vi "Begin.vi"(8 "error in":errorcluster) -> (0 "error out":errorcluster)   [LabVIEW 2018]
doc: "Called before other user functions, this VI can be used to open I/O refnums, load in file data, and do general program initialization. Notice that the <B>error out</B> terminal is simply used for data flow. Wiring it to other structures or subVIs ensures that this VI runs first."
uses:
  <vilib>/Rock Robotics/WPI/DriverStation/WPI_DriverStationRobotMode2.ctl
  <vilib>/Rock Robotics/WPI/Joystick/WPI_JoystickDeviceEnum.ctl
  <vilib>/Rock Robotics/SystemInterfaces/DIO/FPGA_DIOPWMChannel.ctl
  <vilib>/Rock Robotics/WPI/Solenoid/WPI_SolenoidChannel.ctl
  Robot Global Data.vi
  <vilib>/Rock Robotics/Network Tables/NT Write String Array.vi
  <vilib>/Rock Robotics/WPI/RobotDrive/WPI_RobotDriveOpen4MotorWithTalonSRX.vi
  <vilib>/Rock Robotics/WPI/RobotDrive/WPI_RobotDriveOpen4MotorWithVictorSP.vi
  <vilib>/Rock Robotics/WPI/RobotDrive/WPI_RobotDriveOpen2MotorWithVictorSP.vi
  <vilib>/Rock Robotics/WPI/Solenoid/WPI_SolenoidOpenDouble.vi
  <vilib>/Rock Robotics/SystemInterfaces/DIO/FPGA_DIOChannel.ctl
  <vilib>/Rock Robotics/WPI/MotorControl/WPI_MotorControlOpen SPARK.vi
  <vilib>/Rock Robotics/WPI/Counter/WPI_CounterDigitalInputToDigitalSource.vi
  <vilib>/Rock Robotics/WPI/Encoder/WPI_EncoderType.ctl
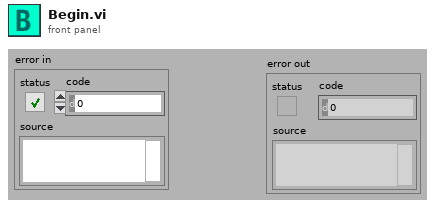
[diagram p1: front panel]
types:
  T1 = typedef "WPI_JoystickDeviceEnum.ctl" = enum16{"USB 0", "USB 1", "USB 2", "USB 3", "USB 4", "USB 5"}
  T2 = typedef "WPI_SolenoidChannel.ctl" = enum8{"Solenoid 0", "Solenoid 1", "Solenoid 2", "Solenoid 3", "Solenoid 4", "Solenoid 5", "Solenoid 6", "Solenoid 7", "Invalid"}
  T3 = typedef "FPGA_DIOPWMChannel.ctl" = enum8{"PWM 0", "PWM 1", "PWM 2", "PWM 3", "PWM 4", "PWM 5", "PWM 6", "PWM 7", "PWM 8", "PWM 9", "PWM MXP 0", "PWM MXP 1", "PWM MXP 2", "PWM MXP 3", "PWM MXP 4", "PWM MXP 5", "PWM MXP 6", "PWM MXP 7", "PWM MXP 8", "PWM MXP 9", "Invalid"}
  T4 = typedef "WPI_DriverStationRobotMode2.ctl" = enum16{"Autonomous Disabled", "Autonomous Enabled", "Teleop Disabled", "Teleop Enabled", "Disconnected", "Finish", "Test Disabled", "Test Enabled", "Emergency Stopped"}
  T5 = typedef "FPGA_DIOChannel.ctl" = enum8{"DIO 0", "DIO 1", "DIO 2", "DIO 3", "DIO 4", "DIO 5", "DIO 6", "DIO 7", "DIO 8", "DIO 9", "DIO MXP 0", "DIO MXP 1", "DIO MXP 2", "DIO MXP 3", "DIO MXP 4", "DIO MXP 5", "DIO MXP 6", "DIO MXP 7", "DIO MXP 8", "DIO MXP 9", "DIO MXP 10", "DIO MXP 11", "DIO MXP 12", "DIO MXP 13", "DIO MXP 14", "DIO MXP 15", "SPI Port CS1", "SPI Port CS2", "SPI Port CS3", "SPI Port MISO", "SPI Port MOSI", "Invalid"}
  T6 = typedef "WPI_CompressorDevRef.ctl" = cluster{"DevStatus":errorcluster, "Pneumatics Control Module":u8}
  T7 = typedef "WPI_DigitalInputDevRef.ctl" = cluster{"DevStatus":errorcluster, "DIO Channel":T5}
  T8 = typedef "WPI_SolenoidDevRef.ctl" = cluster{"DevStatus":errorcluster, "Pneumatics Control Module":u8, "Forward Solenoid Channel":T2, "Reverse Solenoid Channel":T2}
  T9 = typedef "WPI_MotorControlDeviceRef.ctl" = cluster{"DeviceStatus":errorcluster, "Type":T10, "PWM":cluster{"PWM Channel":T3, "DeadBand":T11}, "CAN":cluster{"Device Number":u8, "SetOutput VI Ref":variant, "GetOutput VI Ref":variant, "Enable VI Ref":variant, "Disable VI Ref":variant, "Data":variant}, "Invert":bool, "DIO PWM":cluster{"PWM \"Enable\" Channel":T3, "DIOChannel":T5, "PWM Rate":dbl}}
  T10 = typedef "WPI_MotorControlType.ctl" = enum16{"PWM", "CAN", "DIO PWM"}
  T11 = typedef "WPI_PWMDeadband.ctl" = cluster{"Name":string, "maxPositivePwm":i32, "minPositivePwm":i32, "centerPwm":i32, "maxNegativePwm":i32, "minNegativePwm":i32, "angularRange":u16}
  T12 = typedef "WPI_JoystickDevRef.ctl" = cluster{"Device":T1}
  T13 = typedef "WPI_RobotDriveDevRef.ctl" = cluster{"DevStatus":errorcluster, "Motors[]":T9[], "Square Inputs":bool, "Max Output":dbl}
  T14 = typedef "WPI_EncoderType.ctl" = enum16{"1x", "2x", "4x"}
  T15 = typedef "FPGA_CounterEncoderSourceConvertionLVSourceType.ctl" = cluster{"DevStatus":errorcluster, "AnalogTriggerMode?":bool, "DigitalMode":cluster{"DIO Channel":T16}, "AnalogTriggerMode":cluster{"AnalogTriggerIndex":T17, "OutputType":T18}}
  T16 = typedef "FPGA_DIODigitalSourceChannel.ctl" = enum8{"DIO 0", "DIO 1", "DIO 2", "DIO 3", "DIO 4", "DIO 5", "DIO 6", "DIO 7", "DIO 8", "DIO 9", "DIO MXP 0", "DIO MXP 1", "DIO MXP 2", "DIO MXP 3", "DIO MXP 4", "DIO MXP 5", "DIO MXP 6", "DIO MXP 7", "DIO MXP 8", "DIO MXP 9", "DIO MXP 10", "DIO MXP 11", "DIO MXP 12", "DIO MXP 13", "DIO MXP 14", "DIO MXP 15", "SPI Port CS1", "SPI Port CS2", "SPI Port CS3", "SPI Port MISO", "SPI Port MOSI", "Disabled"}
  T17 = typedef "FPGA_AnalogTriggerIndex.ctl" = enum8{"Trig 0", "Trig 1", "Trig 2", "Trig 3", "Trig 4", "Trig 5", "Trig 6", "Trig 7", "Invalid"}
  T18 = typedef "FPGA_AnalogTriggerOutType.ctl" = enum16{"InWindow", "TriggerState", "Rising", "Falling"}
  T19 = typedef "WPI_EncoderDevRef.ctl" = cluster{"DevStatus":errorcluster, "EncoderIndex":T20, "CounterIndex":T21, "DistancePerCount":dbl, "Decoding Type":T14}
  T20 = typedef "FPGA_EncoderIdx.ctl" = enum8{"Enc 0", "Enc 1", "Enc 2", "Enc 3", "Enc 4", "Enc 5", "Enc 6", "Enc 7", "Invalid"}
  T21 = typedef "FPGA_CounterCtrSystemIndex.ctl" = enum8{"Ctr 0", "Ctr 1", "Ctr 2", "Ctr 3", "Ctr 4", "Ctr 5", "Ctr 6", "Ctr 7", "Invalid"}
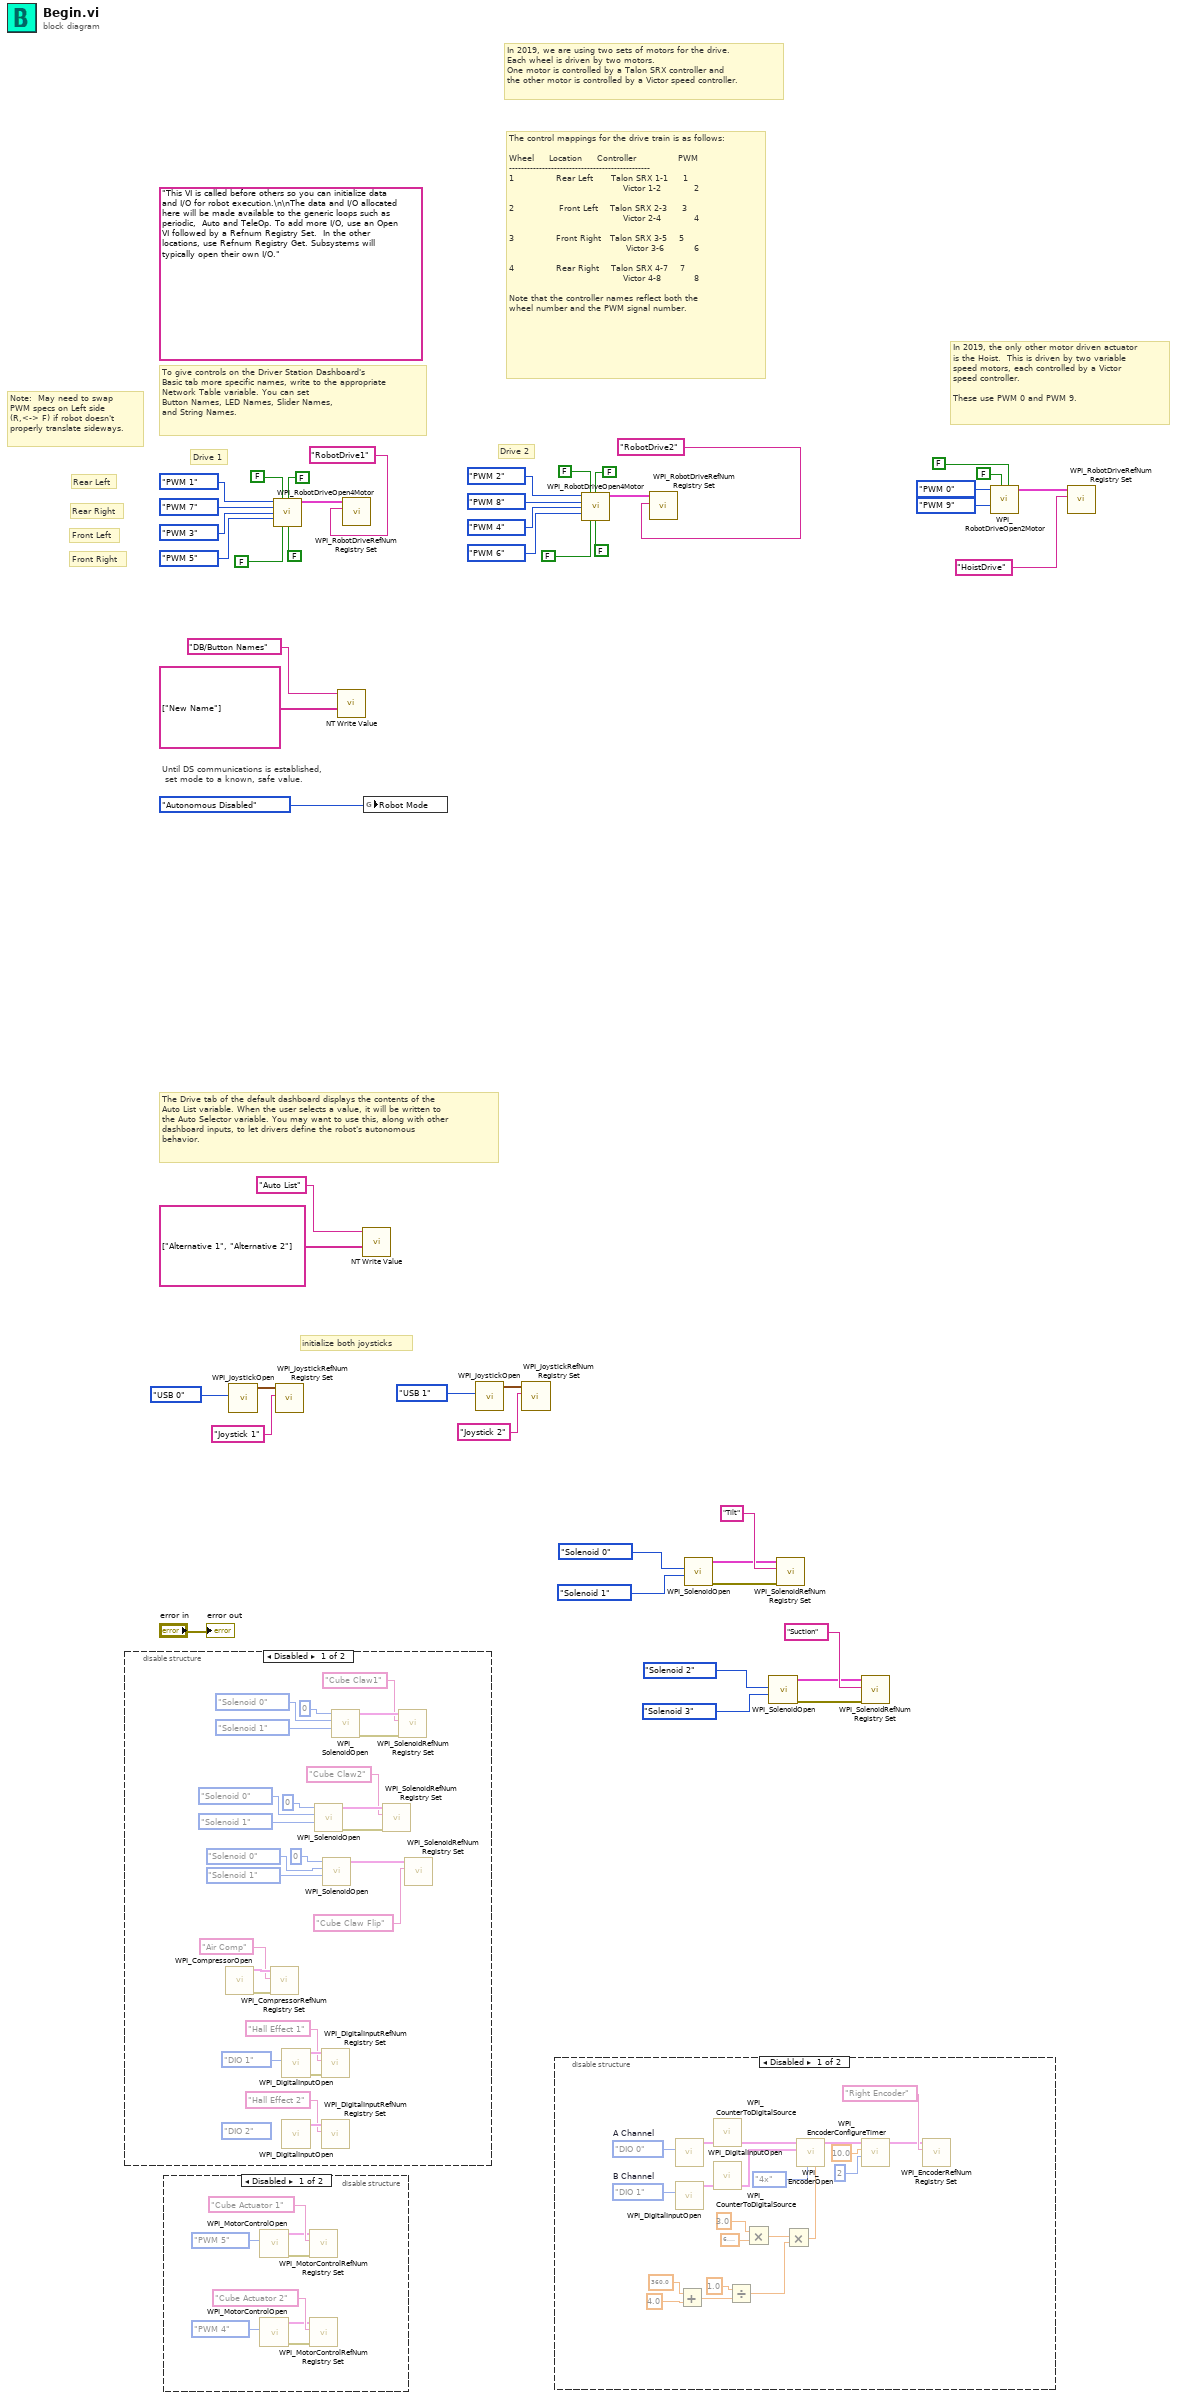
[diagram p0: block diagram]
diagram:
  (unwired) "This VI is called before others so you can initialize data and I/O for robot execution.\n\nThe data and I/O allocated here will be made available to the generic loops such as periodic,  Auto and TeleOp. To add more I/O, use an Open VI followed by a Refnum Registry Set.  In the other locations, use Refnum Registry Get. Subsystems will typically open their own I/O."
  # "In 2019, the only other motor driven actuator\nis the Hoist.  This is driven by two variable\nspeed motors, each controlled by a Victor \nspeed controller.\n\nThese use PWM 0 and PWM 9."
  # "Note:  May need to swap\nPWM specs on Left side \n(R,<-> F) if robot doesn't\nproperly translate sideways."
  # "Front Right"
  # "Front Left"
  # "Rear Left"
  # "Rear Right"
  # "The control mappings for the drive train is as follows:\n\nWheel     Location     Controller              PWM\n-----------------------------------------------\n1              Rear Left      Talon SRX 1-1     1\n                                      Victor 1-2           2\n\n2               Front Left    Talon SRX 2-3     3\n                                      Victor 2-4           4\n\n3              Front Right   Talon SRX 3-5    5\n                                       Victor 3-6          6\n\n4              Rear Right    Talon SRX 4-7    7\n                                      Victor 4-8           8\n\nNote that the controller names reflect both the\nwheel number and the PWM signal number."
  # "Drive 2"
  # "In 2019, we are using two sets of motors for the drive.\nEach wheel is driven by two motors.\nOne motor is controlled by a Talon SRX controller and \nthe other motor is controlled by a Victor speed controller."
  # "Drive 1"
  # "The Drive tab of the default dashboard displays the contents of the\nAuto List variable. When the user selects a value, it will be written to\nthe Auto Selector variable. You may want to use this, along with other\ndashboard inputs, to let drivers define the robot's autonomous\nbehavior."
  # "To give controls on the Driver Station Dashboard's\nBasic tab more specific names, write to the appropriate\nNetwork Table variable. You can set\nButton Names, LED Names, Slider Names,\nand String Names."
  # "initialize both joysticks"
  # "Until DS communications is established,\n set mode to a known, safe value."
  n1 = disable-structure shown="Disabled" {
    frame Disabled {
      (unwired) FPGA_DIOChannel."DIO 2" ("DIO Channel")
      n2 = call <vilib>:"WPI_CompressorOpen.vi"() -> ("CompressorDevRef"=w73:T6, "error out"=w74:errorcluster)  [unwired: 14 in]
      n3 = call <vilib>:"WPI_CompressorRefNum Registry Set.vi"("error in (no error)"=w74, "refnum name"="Air Comp", "CompressorDevRef"=w73) -> ()  [unwired: 7 in, 2 out]
      n4 = call <vilib>:"WPI_DigitalInputOpen.vi"("DIO Channel"=FPGA_DIOChannel."DIO 1") -> ("error out"=w49:errorcluster, "DigitalInputDevRef"=w54:T7)  [unwired: 9 in]
      n5 = call <vilib>:"WPI_DigitalInputOpen.vi"() -> ("DigitalInputDevRef"=w51:T7)  [unwired: 10 in, 1 out]
      n6 = call-poly <vilib>:"WPI_SolenoidOpen.vi"("Reverse Solenoid Channel"=WPI_SolenoidChannel."Solenoid 1", "Forward Solenoid Channel"=WPI_SolenoidChannel."Solenoid 0", "Pneumatics Control Module (0)"=u8 0) -> ("error out"=w64:errorcluster, "SolenoidDevRef"=w65:T8)  [unwired: 7 in]
      n7 = call <vilib>:"WPI_DigitalInputRefNum Registry Set.vi"("error in (no error)"=w49, "refnum name"="Hall Effect 1", "DigitalInputDevRef"=w54) -> ()  [unwired: 7 in, 2 out]
      n8 = call <vilib>:"WPI_DigitalInputRefNum Registry Set.vi"("refnum name"="Hall Effect 2", "DigitalInputDevRef"=w51) -> ()  [unwired: 8 in, 2 out]
      n9 = call-poly <vilib>:"WPI_SolenoidOpen.vi"("Reverse Solenoid Channel"=WPI_SolenoidChannel."Solenoid 1", "Forward Solenoid Channel"=WPI_SolenoidChannel."Solenoid 0", "Pneumatics Control Module (0)"=u8 0) -> ("SolenoidDevRef"=w59:T8)  [unwired: 7 in, 1 out]
      n10 = call-poly <vilib>:"WPI_SolenoidOpen.vi"("Reverse Solenoid Channel"=WPI_SolenoidChannel."Solenoid 1", "Forward Solenoid Channel"=WPI_SolenoidChannel."Solenoid 0", "Pneumatics Control Module (0)"=u8 0) -> ("error out"=w70:errorcluster, "SolenoidDevRef"=w71:T8)  [unwired: 7 in]
      n11 = call <vilib>:"WPI_SolenoidRefNum Registry Set.vi"("error in (no error)"=w64, "refnum name"="Cube Claw2", "SolenoidDevRef"=w65) -> ()  [unwired: 7 in, 2 out]
      n12 = call <vilib>:"WPI_SolenoidRefNum Registry Set.vi"("error in (no error)"=w70, "refnum name"="Cube Claw1", "SolenoidDevRef"=w71) -> ()  [unwired: 7 in, 2 out]
      n13 = call <vilib>:"WPI_SolenoidRefNum Registry Set.vi"("refnum name"="Cube Claw Flip", "SolenoidDevRef"=w59) -> ()  [unwired: 8 in, 2 out]
    }
    frame Enabled {
    }
  }
  n14 = disable-structure shown="Disabled" {
    frame Disabled {
      n15 = call-poly <vilib>:"WPI_MotorControlOpen.vi"("PWM Channel"=FPGA_DIOPWMChannel."PWM 5") -> ("error out"=w78:errorcluster, "MotorControlDeviceRef"=w77:T9)  [unwired: 9 in]
      n16 = call-poly <vilib>:"WPI_MotorControlOpen.vi"("PWM Channel"=FPGA_DIOPWMChannel."PWM 4") -> ("error out"=w80:errorcluster, "MotorControlDeviceRef"=w81:T9)  [unwired: 9 in]
      n17 = call <vilib>:"WPI_MotorControlRefNum Registry Set.vi"("error in (no error)"=w78, "refnum name"="Cube Actuator 1", "MotorControlDevRef"=w77) -> ()  [unwired: 7 in, 2 out]
      n18 = call <vilib>:"WPI_MotorControlRefNum Registry Set.vi"("error in (no error)"=w80, "refnum name"="Cube Actuator 2", "MotorControlDevRef"=w81) -> ()  [unwired: 7 in, 2 out]
    }
    frame Enabled {
    }
  }
  n19 = call <vilib>:"WPI_JoystickOpen.vi"("JoystickDevice"=WPI_JoystickDeviceEnum."USB 0") -> ("JoystickDevRef"=w46:T12)  [unwired: 10 in]
  n20 = call-poly <vilib>:"WPI_RobotDriveOpen4Motor.vi"("Rear Left Motor"=FPGA_DIOPWMChannel."PWM 1", "Rear Left Motor Inverted"=FALSE, "Rear Right Motor Inverted"=FALSE, "Rear Right Motor"=FPGA_DIOPWMChannel."PWM 7", "Front Left Motor"=FPGA_DIOPWMChannel."PWM 3", "Front Right Motor"=FPGA_DIOPWMChannel."PWM 5", "Front Left Motor Inverted"=FALSE, "Front Right Motor Inverted"=FALSE) -> ("RobotDriveDevRef"=w38:T13)  [unwired: 6 in, 1 out]
  n21 = call <vilib>:"WPI_JoystickRefNum Registry Set.vi"("refnum name"="Joystick 1", "JoystickDevRef"=w46) -> ()  [unwired: 8 in, 2 out]
  n22 = call-poly <vilib>:"NT Write Value.vi"("String Array"=string[] ["New Name"], "Name"="DB/Button Names") -> ()  [unwired: 9 in, 1 out]
  n23 = call <vilib>:"WPI_RobotDriveRefNum Registry Set.vi"("refnum name"="RobotDrive1", "RobotDriveDevRef"=w38) -> ()  [unwired: 8 in, 2 out]
  n24 = call-poly <vilib>:"NT Write Value.vi"("String Array"=string[] ["Alternative 1", "Alternative 2"], "Name"="Auto List") -> ()  [unwired: 9 in, 1 out]
  n25 = global write "Robot Global Data.vi" "Robot Mode"(WPI_DriverStationRobotMode2."Autonomous Disabled" ("Robot Mode")) -> ()
  n26 = call <vilib>:"WPI_JoystickOpen.vi"("JoystickDevice"=WPI_JoystickDeviceEnum."USB 1") -> ("JoystickDevRef"=w2:T12)  [unwired: 10 in]
  n27 = call <vilib>:"WPI_JoystickRefNum Registry Set.vi"("refnum name"="Joystick 2", "JoystickDevRef"=w2) -> ()  [unwired: 8 in, 2 out]
  n28 = disable-structure shown="Disabled" {
    frame Disabled {
      w103 = FPGA_DIOChannel."DIO 1"  # B Channel
      w102 = FPGA_DIOChannel."DIO 0"  # A Channel
      n29 = call <vilib>:"WPI_DigitalInputOpen.vi"("DIO Channel"=w102) -> ("DigitalInputDevRef"=w99:T7)  [unwired: 1 in, 9 out]
      n30 = call <vilib>:"WPI_DigitalInputOpen.vi"("DIO Channel"=w103) -> ("DigitalInputDevRef"=w100:T7)  [unwired: 1 in, 9 out]
      n31 = Add(x=360.0, y=4.0) -> (x+y=w88:dbl)
      n32 = call-poly <vilib>:"WPI_CounterToDigitalSource.vi"("DigitalInputDevRef"=w99) -> ("Digital Source"=w98:T15)  [unwired: 6 out]
      n33 = call-poly <vilib>:"WPI_CounterToDigitalSource.vi"("DigitalInputDevRef"=w100) -> ("Digital Source"=w101:T15)  [unwired: 6 out]
      n34 = Divide(x=1.0, y=w88) -> (x/y=w90:dbl)
      n35 = Multiply(x=3.0, y=6.283185307179586) -> (x*y=w91:dbl)
      n36 = Multiply(x=w91, y=w90) -> (x*y=w83:dbl)
      n37 = call <vilib>:"WPI_EncoderOpen.vi"("DistancePerCount"=w83, "Decoding Type"=WPI_EncoderType."4x", "BSource"=w101, "ASource"=w98) -> ("EncoderDevRef"=w96:T19)  [unwired: 4 in, 3 out]
      n38 = call <vilib>:"WPI_EncoderConfigureTimer.vi"("Number Samples to Average"=u8 2, "Minimum Rate"=10.0, "EncoderDevRef"=w96) -> ("EncoderDevRef"=w92:T19)  [unwired: 7 in, 1 out]
      n39 = call <vilib>:"WPI_EncoderRefNum Registry Set.vi"("refnum name"="Right Encoder", "EncoderDevRef"=w92) -> ()  [unwired: 8 in, 2 out]
    }
    frame Enabled {
    }
  }
  n40 = call-poly <vilib>:"WPI_RobotDriveOpen4Motor.vi"("Rear Left Motor"=FPGA_DIOPWMChannel."PWM 2", "Rear Left Motor Inverted"=FALSE, "Rear Right Motor Inverted"=FALSE, "Rear Right Motor"=FPGA_DIOPWMChannel."PWM 8", "Front Left Motor"=FPGA_DIOPWMChannel."PWM 4", "Front Right Motor"=FPGA_DIOPWMChannel."PWM 6", "Front Left Motor Inverted"=FALSE, "Front Right Motor Inverted"=FALSE) -> ("RobotDriveDevRef"=w28:T13)  [unwired: 6 in, 1 out]
  n41 = call <vilib>:"WPI_RobotDriveRefNum Registry Set.vi"("refnum name"="RobotDrive2", "RobotDriveDevRef"=w28) -> ()  [unwired: 8 in, 2 out]
  n42 = call-poly <vilib>:"WPI_SolenoidOpen.vi"("Reverse Solenoid Channel"=WPI_SolenoidChannel."Solenoid 1", "Forward Solenoid Channel"=WPI_SolenoidChannel."Solenoid 0") -> ("error out"=w11:errorcluster, "SolenoidDevRef"=w12:T8)  [unwired: 8 in]
  n43 = call-poly <vilib>:"WPI_SolenoidOpen.vi"("Reverse Solenoid Channel"=WPI_SolenoidChannel."Solenoid 3", "Forward Solenoid Channel"=WPI_SolenoidChannel."Solenoid 2") -> ("error out"=w6:errorcluster, "SolenoidDevRef"=w7:T8)  [unwired: 8 in]
  n44 = call <vilib>:"WPI_SolenoidRefNum Registry Set.vi"("error in (no error)"=w11, "refnum name"="Tilt", "SolenoidDevRef"=w12) -> ()  [unwired: 7 in, 2 out]
  n45 = call <vilib>:"WPI_SolenoidRefNum Registry Set.vi"("error in (no error)"=w6, "refnum name"="Suction", "SolenoidDevRef"=w7) -> ()  [unwired: 7 in, 2 out]
  n46 = call-poly <vilib>:"WPI_RobotDriveOpen2Motor.vi"("Right Motor Inverted"=FALSE, "Left Motor Inverted"=FALSE, "Right Motor"=FPGA_DIOPWMChannel."PWM 9", "Left Motor"=FPGA_DIOPWMChannel."PWM 0") -> ("RobotDriveDevRef"=w15:T13)  [unwired: 6 in, 1 out]
  n47 = call <vilib>:"WPI_RobotDriveRefNum Registry Set.vi"("refnum name"="HoistDrive", "RobotDriveDevRef"=w15) -> ()  [unwired: 8 in, 2 out]
  "error out" <- "error in"
